vi "GT Get Ext Do Value.vi"(8 "error in (no error)":errorcluster caption="错误输入（无错误）", 9 "pValue":u16, 10 "mdl":i16, 11 "cardNum":i16) -> (0 "error out":errorcluster caption="错误输出", 1 "pValue out":u16, 3 "function return":i16)   [LabVIEW 2014, in "gts.lvlib"]
doc: "GT_API GT_GetExtDoValue(short cardNum,short mdl,unsigned short *pValue);"
uses:
  gts.lvlib
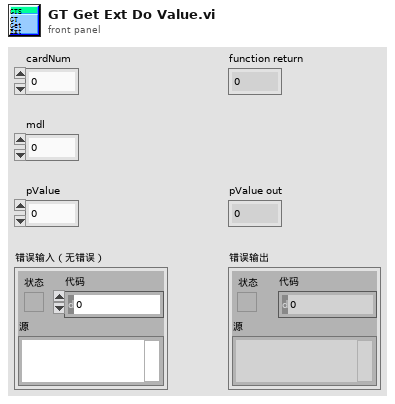
[diagram p1: front panel]
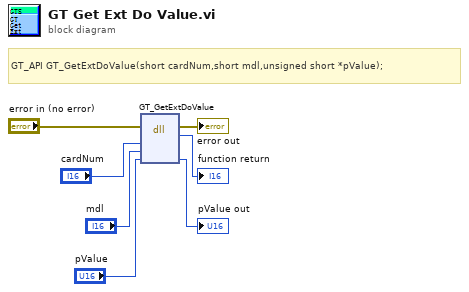
[diagram p0: block diagram]
diagram:
  # "GT_API GT_GetExtDoValue(short cardNum,short mdl,unsigned short *pValue);"
  n1 = dll-call lib="PTH2habs D固高科技资料GTS控制卡GTS卡18年上半年资料dllVC32bit\nmulti_cardgts.*" fn="GT_GetExtDoValue"(error in="error in (no error)", "cardNum"="cardNum", "mdl"="mdl", "pValue"="pValue") -> (error out=→"error out":errorcluster, →"function return":i16, "pValue"=→"pValue out":u16)  [unwired: 4 in, 1 out]
